vi "Read Val.vi"(8 "error in (no error)":errorcluster, 11 "DBL STEP in":refnum<class "DBL STEP.lvclass">) -> (0 "error out":errorcluster, 2 "Val":dbl, 3 "DBL STEP out":refnum<class "DBL STEP.lvclass">)   [LabVIEW 2014, in "DBL STEP.lvlib" / "DBL STEP.lvclass"]
uses:
  DBL STEP.lvclass
  DBL STEP.lvclass/DBL STEP.ctl
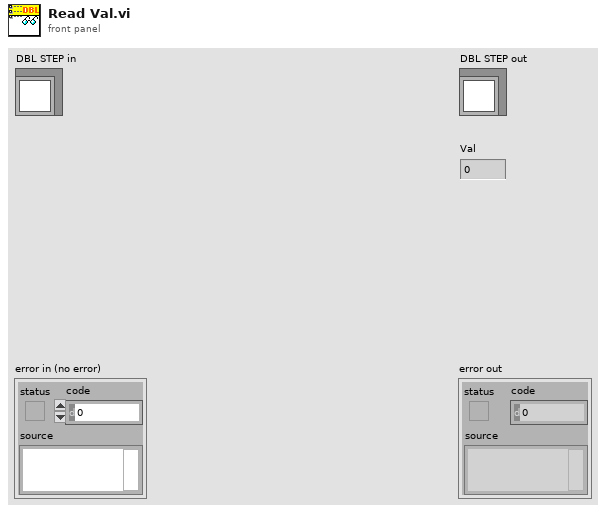
[diagram p1: front panel]
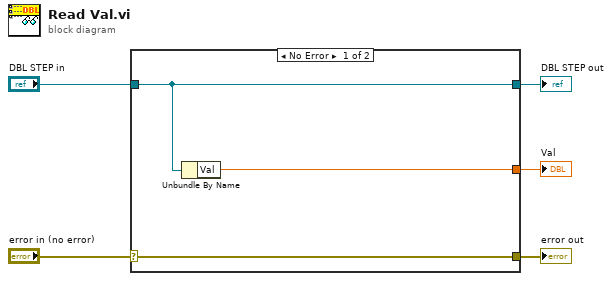
[diagram p0: block diagram]
diagram:
  n1 = case shown="No Error" "error in (no error)" {
    selector: "error in (no error)" -> [w8 w9]
    tunnel: [w8 w9] -> w4
    tunnel: [w7 w10] -> w2
    tunnel: "DBL STEP in" -> [w7 w10]
    tunnel: [w6 _] -> w1
    frame No Error {
      n2 = Unbundle By Name(w7) -> ("Val"=w6:dbl)
    }
    frame Error {
    }
  }
  "error out" <- w4
  "DBL STEP out" <- w2
  "Val" <- w1
